vi "Write Data.vi"(6 "chip select (1st chip)":enum16{"1st chip", "2nd chip"}(ring), 8 "error in (no error)":errorcluster, 10 "character code":u8=97 format="%.0x", 11 "LCD in":u32) -> (0 "error out":errorcluster, 3 "LCD out":u32)   [LabVIEW 2015, in "HD44780 FPGA.lvlib"]
doc: "Writes data to character LCD devices. After you call this VI, the address increases or decreases by one according to the entry mode. The entry mode also determines the display shift."
uses:
  <vilib>/EmbeddedDisplay/Hitachi HD44780/FPGA/HD44780 FPGA.lvlib
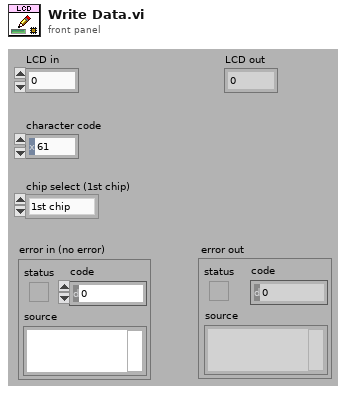
[diagram p1: front panel]
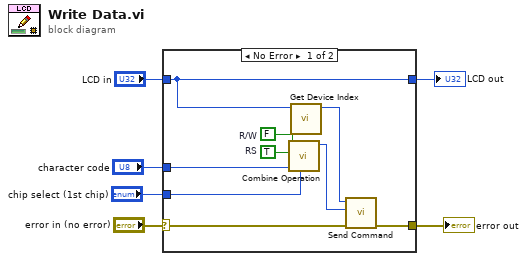
[diagram p0: block diagram]
diagram:
  n1 = case shown="No Error" "error in (no error)" {
    selector: "error in (no error)" -> [w14 w17]
    tunnel: [w13 w17] -> w5
    tunnel: "character code" -> [w12 _]
    tunnel: "chip select (1st chip)" -> [w10 _]
    tunnel: "LCD in" -> [w7 w16]
    tunnel: [w7 w16] -> w1
    frame No Error {
      w15 = FALSE  # R/W
      w11 = TRUE  # RS
      n2 = call <vilib>:"Combine Operation.vi"("chip select  (1st chip)"=w10, "cmd/data (0)"=w12, "RS"=w11, "R/W"=w15) -> ("output"=w8:u32)  [unwired: 7 in]
      n3 = call <vilib>:"Get Device Index.vi"("LCD in"=w7) -> ("device index"=w9:i8)  [unwired: 10 in]
      n4 = call <vilib>:"Send Command.vi"("error in (no error)"=w14, "operation"=w8, "device index"=w9) -> ("error out"=w13:errorcluster)  [unwired: 6 in, 2 out]
    }
    frame Error {
    }
  }
  "error out" <- w5
  "LCD out" <- w1
